vi "get images.vi"(8 "error in (no error)":errorcluster, 11 "MapSite in":refnum<class "MapSite.lvclass">) -> (0 "error out":errorcluster, 2 "images":T1[](array[typedef]), 3 "MapSite out":refnum<class "MapSite.lvclass">)   [LabVIEW 2016, in "MapSite.lvclass"]
uses:
  MapSite.lvclass
  <vilib>/picture/picture.llb/imagedata.ctl
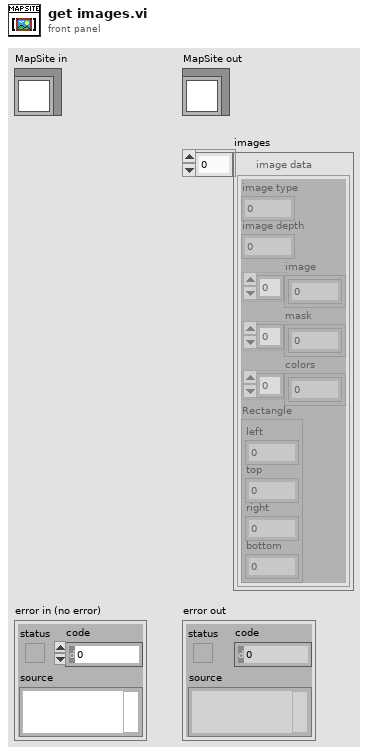
[diagram p1: front panel]
types:
  T1 = typedef "imagedata.ctl" = cluster{"image type":i32, "image depth":i32, "image":u8[], "mask":u8[], "colors":u32[], "Rectangle":cluster{"left":i16, "top":i16, "right":i16, "bottom":i16}}
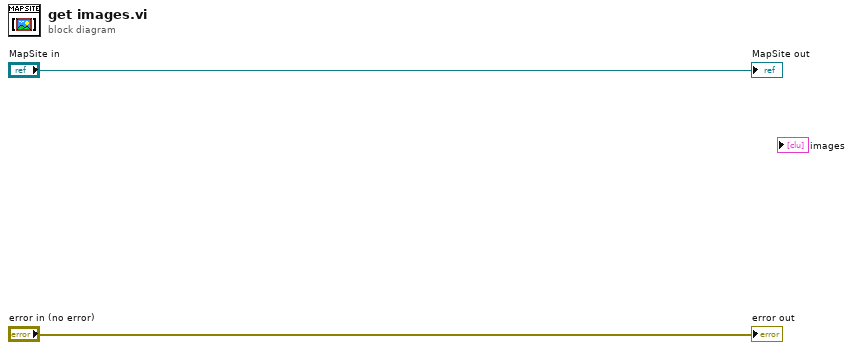
[diagram p0: block diagram]
diagram:
  "error out" <- "error in (no error)"
  "MapSite out" <- "MapSite in"
